vi "Thruster.vi"   [LabVIEW 2014, in "Thruster.lvclass"]
uses:
  Thruster.lvclass
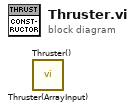
[diagram p0: block diagram]
diagram:
  n1 = call "Thruster(ArrayInput).vi"() -> ()  [unwired: 11 in, 1 out]
  n2 = call "Thruster().vi"() -> ()  [unwired: 11 in, 1 out]
